vi "Actor Core.vi"(8 "error in":errorcluster, 11 "CI Mediator in":refnum<class "CI Mediator.lvclass">) -> (0 "error out":errorcluster, 3 "Actor out":refnum<class "Actor.lvclass">)   [LabVIEW 2014, in "CI Mediator.lvlib" / "CI Mediator.lvclass"]
doc: "(<B>Filename</B>: Actor Framework.lvlib:Actor.lvclass:Actor Core.vi)\n\nReceives messages to the actor, reacts to them, and initiates any error handling that may shut the actor down.\n\nDescendant classes may override this VI to append parallel tasks for the actor to complete while it handles messages. Overrides use the Call Parent Method node."
uses:
  CI Mediator.lvclass
  <vilib>/ActorFramework/Actor/Actor.lvclass
  Controls/Executor Status - STYP.ctl
  <vilib>/ActorFramework/Actor/Actor.lvclass/Actor.ctl
  <vilib>/ActorFramework/Message Enqueuer/Message Enqueuer.lvclass/Message Enqueuer.ctl
  CI Mediator.lvclass/CI Mediator.ctl
  <vilib>/ActorFramework/Message Enqueuer/Init from Existing Queue.vi
  <vilib>/ActorFramework/Message Enqueuer/Enqueue.vi
  <vilib>/ActorFramework/Message Priority Queue/Priority Enqueue.vi
  <vilib>/ActorFramework/Message Enqueuer/Message Enqueuer.lvclass
  CI Mediator Messages/Exit Msg/Exit Msg.lvclass
  Classes/Executor/Executor.lvclass
panel:
  out "Display Message":string
  in  "Exit":bool
  out "Uptime:":dbl format="%<%H:%M:%S>t"
  out "Executors":T1[](array[typedef])
  out "Ball Cluster":T2
  # "LabVIEW CI Service"
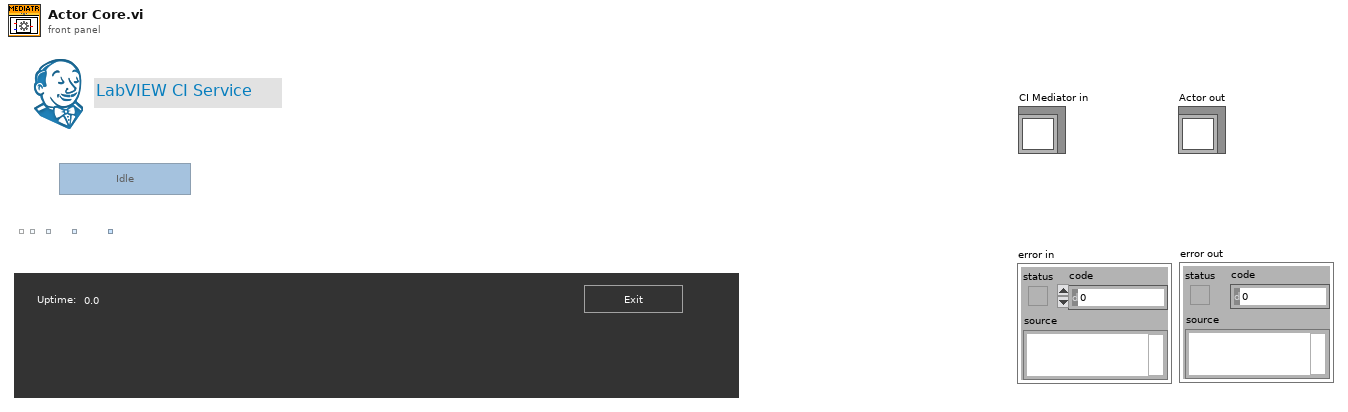
[diagram p1: front panel]
types:
  T1 = typedef "Executor Status - STYP.ctl" = cluster{"Executor Name":string, "Status":bool}
  T2 = cluster{"Boolean":bool, "Boolean 2":bool, "Boolean 3":bool, "Boolean 4":bool, "Boolean 5":bool, "Boolean 6":bool}
  T3 = enum32{"Invalid", "Standard", "Closed", "Hidden", "Minimized", "Maximized"}
  T4 = cluster{"Stop":refnum<user-event>, "Executor Status":refnum<user-event>}
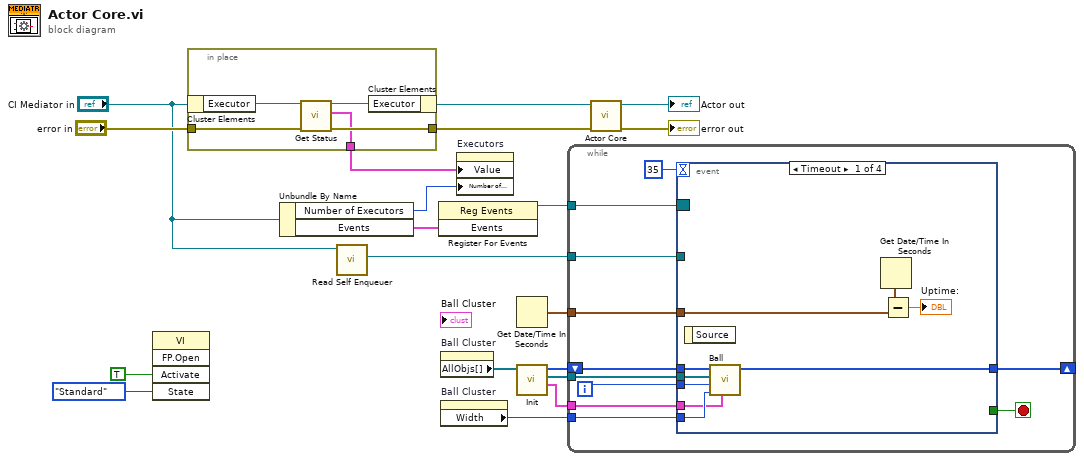
[diagram p0: block diagram]
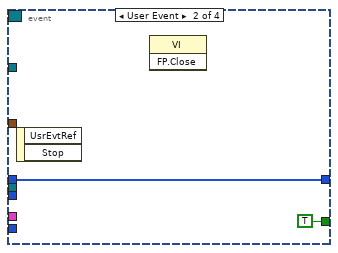
[diagram p2: hidden frame]
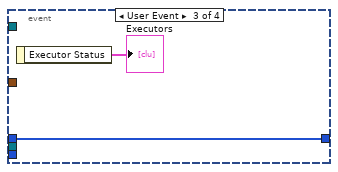
[diagram p3: hidden frame]
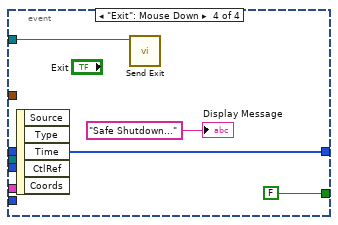
[diagram p4: hidden frame]
diagram:
  n1 = invoke class="VI" method="FP.Open"("Activate"=TRUE ("Activate?"), "State"=T3."Standard") -> ()  [unwired: 3 in, 5 out]
  n2 = in-place {
    in-place-border: "error in" -> [w24]
    in-place-border: [w23] -> w5
    in-place-border: [w20] -> w2
    n3 = in-place-cluster #1("CI Mediator in") -> ("Executor"=w22:refnum<class "Executor.lvclass">)
    n4 = call "Get Status.vi"("error in (no error)"=w24, "Executor Reference"=w22) -> ("error out"=w23:errorcluster, "Status[]"=w20:T1[], "Executor Reference"=w21:refnum<class "Executor.lvclass">)  [unwired: 6 in, 1 out]
    n5 = in-place-cluster #1("Executor"=w21) -> (w3:refnum<class "CI Mediator.lvclass">)
  }
  n6 = Unbundle By Name("CI Mediator in") -> ("Number of Executors"=w7:i32, "Events"=w12:T4)
  n7 = call <vilib>:"Read Self Enqueuer.vi"("Actor"="CI Mediator in") -> ("Self Enqueuer"=w10:refnum<class "Message Enqueuer.lvclass">)  [unwired: 10 in]
  n8 = register-events(w12) -> (reference out=w11:refnum<event-registration>)  [unwired: 2 in, 1 out]
  n9 = property on="Ball Cluster" class="Clust (strict)"() -> ("AllObjs[]"=w17:refnum<vi>[])  [unwired: 2 in, 2 out]
  n10 = property on="Ball Cluster" class="Clust (strict)"() -> ("Width"=w14:u32)  [unwired: 2 in, 2 out]
  n11 = property on="Executors" class="Arr (strict)"("Value"=w2, "Number of Columns"=w7) -> ()  [unwired: 2 in, 2 out]
  n12 = Get Date/Time In Seconds() -> (seconds since 1Jan1904=w13:timestamp)
  n13 = call "Init.vi"("AllObjs[]"=w17) -> ("Ball Ref"=w1:cluster{refnum<vi>, "PaneColor":u32}[], "Array 2"=w15:refnum<vi>[], "Array"=w16:i32[])  [unwired: 8 out]
  n14 = while {
    shift-right: [w33] -> _
    shift-left: w16 -> [w34]
    tunnel: w15 -> [w32]
    tunnel: w14 -> [w31]
    tunnel: w13 -> [w30]
    tunnel: w11 -> [w27]
    tunnel: w10 -> [w26]
    tunnel: w1 -> [w25]
    i -> [w35]
    stop <- w28 stop-if-true
    n15 = event shown="[0] Timeout" {
      selector: w27 -> [_ _ _ _]
      dyn-events: _ -> [_ _ _ _]
      timeout: 35 -> [_ _ _ _]
      tunnel: w35 -> [w44 _ _ _]
      tunnel: w34 -> [w43 w45 w47 w49]
      tunnel: [w42 w45 w47 w49] -> w33
      tunnel: w32 -> [w41 _ _ _]
      tunnel: w31 -> [w40 _ _ _]
      tunnel: w30 -> [w38 _ _ _]
      tunnel: [_ TRUE _ FALSE] -> w28
      tunnel: w26 -> [_ _ _ w51]
      tunnel: w25 -> [w36 _ _ _]
      event Timeout {
        n16 = event-data() -> ()  [unwired: 1 in, 1 out]
        n17 = call "Ball.vi"("Ball Ref"=w36, "Cluster width"=w40, "Main Loop Iterations"=w44, "Ball Refs"=w41, "Positions In"=w43) -> ("Positions Out"=w42:i32[])  [unwired: 6 in]
        n18 = Get Date/Time In Seconds() -> (seconds since 1Jan1904=w39:timestamp)
        n19 = Subtract(x=w39, y=w38) -> (x-y=→"Uptime:":dbl)
      }
      event User Event {
        n20 = event-data() -> ()  [unwired: 1 in, 2 out]
        n21 = invoke class="VI" method="FP.Close"() -> ()  [unwired: 3 in, 3 out]
      }
      event User Event {
        n22 = event-data() -> ("Executor Status"=→"Executors":T1[])  [unwired: 1 in]
      }
      event "Exit": Mouse Down {
        n23 = event-data() -> ()  [unwired: 1 in, 5 out]
        n24 = call "Send Exit.vi"("Message Enqueuer"=w51) -> ()  [unwired: 9 in, 2 out]
        "Display Message" <- "Safe Shutdown..." ("Display Message")
      }
    }
  }
  n25 = call-parent "Actor Core.vi"("error in"=w5, "Actor in"=w3) -> ("error out"=→"error out":errorcluster, "Actor out"=→"Actor out":refnum<class "Actor.lvclass">)  [unwired: 8 in]
